vi "Set CCD configuration.vi"(8 "error in (no error)":errorcluster, 11 "CCD in":refnum<class "CCD.lvclass">) -> (0 "error out":errorcluster, 3 "CCD out":refnum<class "CCD.lvclass">)   [LabVIEW 2018, in "CCD.lvclass"]
uses:
  CCD.lvclass
  CCD.lvclass/CCD.ctl
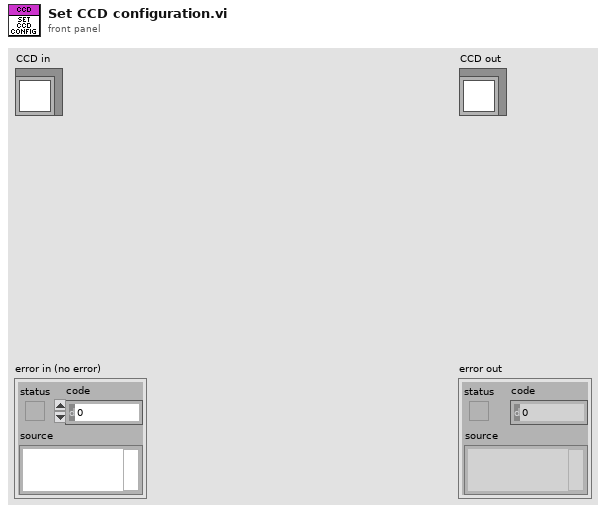
[diagram p1: front panel]
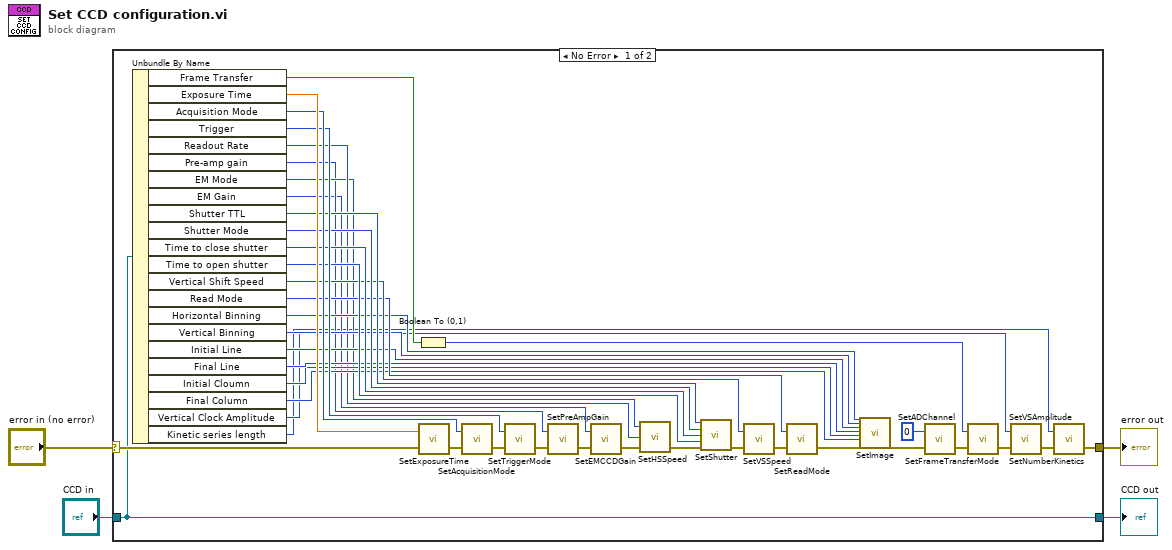
[diagram p0: block diagram]
diagram:
  n1 = case shown="No Error" "error in (no error)" {
    selector: "error in (no error)" -> [w21 w46]
    tunnel: [w5 w46] -> w2
    tunnel: [w6 w45] -> w1
    tunnel: "CCD in" -> [w6 w45]
    frame No Error {
      n2 = Unbundle By Name(w6) -> ("Frame Transfer"=w12:bool, "Exposure Time"=w43:dbl, "Acquisition Mode"=w42:u8, "Trigger"=w41:u8, "Readout Rate"=w20:u8, "Pre-amp gain"=w17:u8, "EM Mode"=w19:u8, "EM Gain"=w14:u32, "Shutter TTL"=w40:u8, "Shutter Mode"=w39:u8, "Time to close shutter"=w38:u16, "Time to open shutter"=w37:u16, "Vertical Shift Speed"=w36:u8, "Read Mode"=w35:u8, "Horizontal Binning"=w30:u16, "Vertical Binning"=w29:u16, "Initial Line"=w28:u16, "Final Line"=w27:u16, "Initial Cloumn"=w26:u16, "Final Column"=w25:u16, "Vertical Clock Amplitude"=w9:u8, "Kinetic series length"=w8:u32)
      n3 = Boolean To (0,1)(Boolean=w12) -> (0, 1=w11:i16)
      n4 = call <userlib>:"SetExposureTime.vi"("error in (no error)"=w21, "time"=w43) -> ("error out"=w34:errorcluster)  [unwired: 1 out]
      n5 = call <userlib>:"SetAcquisitionMode.vi"("error in (no error)"=w34, "mode"=w42) -> ("error out"=w33:errorcluster)  [unwired: 1 out]
      n6 = call <userlib>:"SetTriggerMode.vi"("error in (no error)"=w33, "mode"=w41) -> ("error out"=w18:errorcluster)  [unwired: 1 out]
      n7 = call <userlib>:"SetPreAmpGain.vi"("error in (no error)"=w18, "index"=w17) -> ("error out"=w15:errorcluster)  [unwired: 1 out]
      n8 = call <userlib>:"SetEMCCDGain.vi"("error in (no error)"=w15, "gain"=w14) -> ("error out"=w16:errorcluster)  [unwired: 1 out]
      n9 = call <userlib>:"SetHSSpeed.vi"("error in (no error)"=w16, "index"=w20, "type"=w19) -> ("error out"=w22:errorcluster)  [unwired: 1 in, 1 out]
      n10 = call <userlib>:"SetShutter.vi"("type"=w40, "mode"=w39, "closingtime"=w38, "openingtime"=w37, "error in (no error)"=w22) -> ("error out"=w32:errorcluster)  [unwired: 9 in, 1 out]
      n11 = call <userlib>:"SetVSSpeed.vi"("error in (no error)"=w32, "index"=w36) -> ("error out"=w31:errorcluster)  [unwired: 1 out]
      n12 = call <userlib>:"SetReadMode.vi"("error in (no error)"=w31, "mode"=w35) -> ("error out"=w24:errorcluster)  [unwired: 1 out]
      n13 = call <userlib>:"SetImage.vi"("hbin"=w30, "vbin"=w29, "hstart"=w28, "hend"=w27, "vstart"=w26, "vend"=w25, "error in (no error)"=w24) -> ("error out"=w23:errorcluster)  [unwired: 19 in, 1 out]
      n14 = call <userlib>:"SetADChannel.vi"("error in (no error)"=w23, "channel"=0) -> ("error out"=w13:errorcluster)  [unwired: 1 out]
      n15 = call <userlib>:"SetFrameTransferMode.vi"("error in (no error)"=w13, "mode"=w11) -> ("error out"=w10:errorcluster)  [unwired: 1 out]
      n16 = call <userlib>:"SetVSAmplitude.vi"("error in (no error)"=w10, "amplitude"=w9) -> ("error out"=w7:errorcluster)  [unwired: 1 out]
      n17 = call <userlib>:"SetNumberKinetics.vi"("error in (no error)"=w7, "number"=w8) -> ("error out"=w5:errorcluster)  [unwired: 1 out]
    }
    frame Error {
    }
  }
  "error out" <- w2
  "CCD out" <- w1
